vi "MotorEndLimitSwitch.vi"(9 "MotorCommand":dbl format="%#_13g", 10 "ReverseLimit":bool=TRUE, 11 "ForwardLimit":bool=TRUE) -> (1 "MotorCommand Out":dbl)   [LabVIEW 2015]
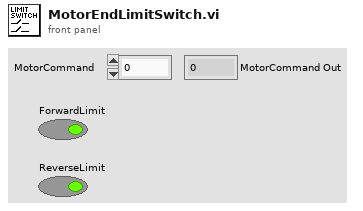
[diagram p1: front panel]
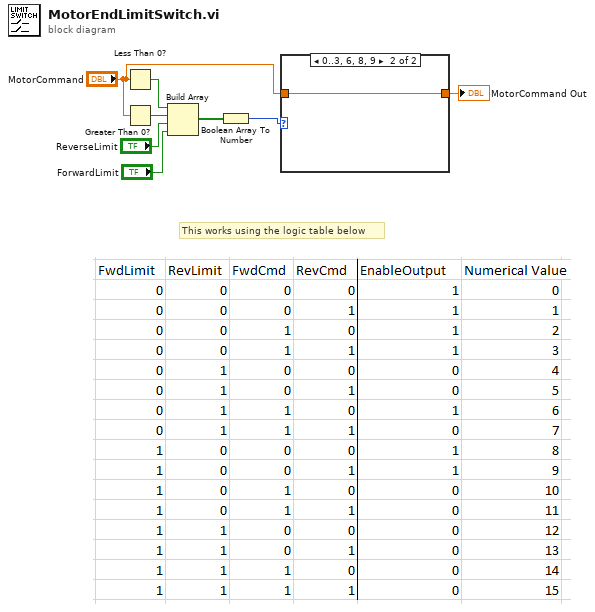
[diagram p0: block diagram]
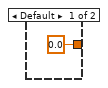
[diagram p2: hidden frame]
diagram:
  # "This works using the logic table below"
  n1 = Less Than 0?(x="MotorCommand") -> (x < 0?=w8:bool)
  n2 = Greater Than 0?(x="MotorCommand") -> (x > 0?=w7:bool)
  n3 = Build Array(w8, w7, "ReverseLimit", "ForwardLimit") -> (w4:bool[])
  n4 = Boolean Array To Number(Boolean array=w4) -> (number=w3:u32)
  n5 = case shown="0..3, 6, 8, 9" w3 {
    tunnel: "MotorCommand" -> [_ w10]
    tunnel: [0.0 ("MotorCommand") w10] -> w1
    frame Default {
    }
    frame 0..3, 6, 8, 9 {
    }
  }
  "MotorCommand Out" <- w1
